vi "10-Tap 8-Bit Camera with DRAM (Host).vi"() -> ()   [LabVIEW 2014]
doc: "This is the host VI for the 10-Tap 8-Bit Camera with DRAM example. This example demonstrates how to acquire images from a 10-tap, 8-bit, extended configuration, Camera Link camera and display the images on the host. This example supports area scan and line scan cameras for both continuous and finite acquisitions.\n\nThis example also demonstrates the use of DRAM as a frame buffer for very high speed acquisitions. Data packing and flow-control are also employed to maximize use of the available DRAM and FIFOs in terms of both memory space and performance.\n\nAdditionally, the example demonstrates the serial server, which allows third-party camera configuration utilities to communicate with the camera using the Camera Link serial interface while this VI is running."
uses:
  <vilib>/userdefined/High Color/nirio_resource_hc.ctl
  <vilib>/FPGAPlugInAG/PCIe-1473R/niLvFpga_Open_PCIe-1473R.vi
  <vilib>/rvi/interface/common/dynamic/niFpgaDynamicAddResources.vi
  <vilib>/FPGAPlugInAG/Dynamic/niLvFpga_Reset_Dynamic.vi
  <vilib>/Utility/error.llb/Error Cluster From Error Code.vi
  <vilib>/rvi/errors/niLvFpgaAdjustHostInterfaceError.vi
  <vilib>/FPGAPlugInAG/Dynamic/niLvFpga_Run_Dynamic.vi
  <vilib>/rvi/interface/common/niFpgaWaitOnOcc.vi
  <vilib>/DAQmx/write.llb/DAQmx Write (Analog DBL 1Chan 1Samp).vi
  <vilib>/FPGAPlugInAG/Dynamic/niLvFpga_Close_Dynamic.vi
  <vilib>/rvi/interface/nirviOpenFPGA/nirviOpenFPGA.xnode
  FPGA Bitfiles/10-Tap8-bitCamer_FPGATarget_10-Tap8-bitCamer_C490DC32.lvbitx
  <vilib>/rvi/interface/nirviMethod/nirviMethod.xnode
  <vilib>/rvi/interface/nirviReadWriteControl/nirviReadWriteControl.xnode
  <vilib>/rvi/interface/nirviCloseFPGA/nirviCloseFPGA.xnode
  <vilib>/rvi/interface/Simulation/niFpgaSimulationCallBeginRW.vi
  <vilib>/rvi/errors/niLvFpgaMergeErrorWithErrorCode.vi
  NiFpgaLv.dll
  <vilib>/FPGAPlugInAG/Dynamic/niLvFpga_ConfigureFifo_Dynamic.vi
  <vilib>/FPGAPlugInAG/Dynamic/niLvFpga_StartFifo_Dynamic.vi
  <vilib>/FPGAPlugInAG/Dynamic/niLvFpga_ReadFifo_Dynamic.vi
  fish tracking dll/labview/find_fish_position.lvlib
  fish tracking dll/bin/find_fish_position.dll
panel:
  in  "Bin Threshold":i32=30
  in  "Axis Speed":dbl=50.0
  in  "Joystick":bool
  in  "Track":bool
  out "FISH_FOUND":bool
  in  "Bkg Image Path (must be the same size as the grabbed image)":path=path "C:/Users/Elizabeth/Desktop/bck_fish.png"
  in  "shift":i32
  in  "ROI_height":i32=180
  in  "ROI_witdth":i32=180
  out "Centroid":cluster{"y":i32, "x":i32}
  in  "SpeedFactor":dbl=1.0
  in  "offset":dbl(slide)=172.02643171806167 scale=150.0..250.0
  in  "Y_Target":dbl=219.0
  in  "X_Target":dbl=211.0
  out "TimeDelay":dbl=0.003333078930154443
  in  "setROI":bool=TRUE
  out "DstImageOpenCV":T1(plugin-control)
  in  "Esize_open":i32(slide)=4 scale=3.0..10.0
  in  "Esize_close":i32(slide)=4 scale=3.0..10.0
  in  "DMA Buffer Size\n(In Images)":u32=64 caption="DMA Buffer Size"
  in  "Signal Mapping":T2(ring)=enum."Basler 10-tap"
  out "Acq In Progress":bool=TRUE
  in  "Line Scan":bool
  in  "Frames To Acquire":u32 caption="Frames To Acquire\n(0 = infinite)"
  in  "Cancel":bool
  out "Acq'd Frame Width":u32=480
  in  "Stopped":bool=TRUE
  in  "RIO Device":T3="RIO0"
  out "DMA Write Timeout":bool
  in  "Start Serial Server":bool=TRUE
  out "Frames Acq'd":u32=128789
  out "Acq'd Frame Height":u32=400
  in  "Acquire":bool
  in  "Stop":bool
  in  "Image Height":u32=400 max=65535
  in  "Image Width":u32=480 max=65535 step=40
  out "Initialized":bool
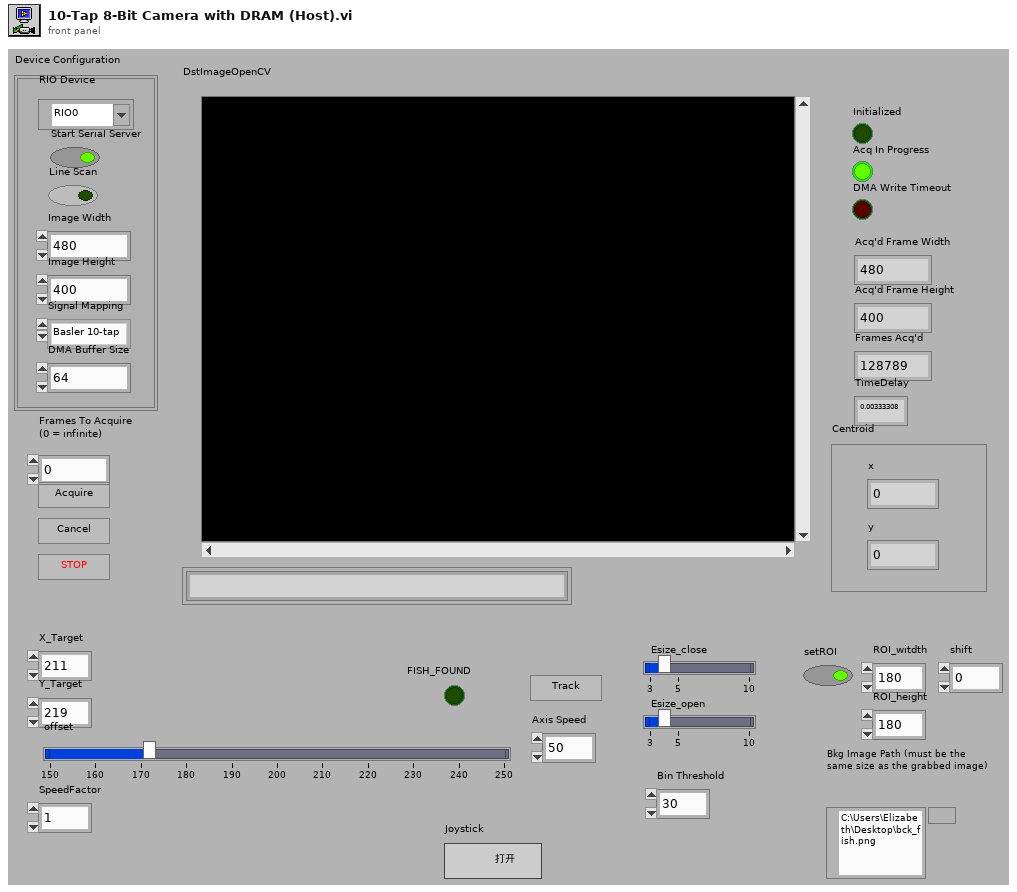
[diagram p1: front panel]
types:
  T1 = typedef "IMAQ Image.ctl" = refnum<image>
  T2 = enum8{"Standard", "Basler 10-tap", "Vosskühler 10-tap"}
  T3 = typedef "nirio_resource_hc.ctl" = tag
  T4 = typedef "Image Type" = u32
  T5 = enum16{"big-endian, network order", "native, host order", "little-endian"}
  T6 = enum32{"Invalid", "Standard", "Closed", "Hidden", "Minimized", "Maximized"}
  T7 = enum32{"Map Pixel Pointer", "Unmap Pixel Pointer", "Get Pixels Infos"}
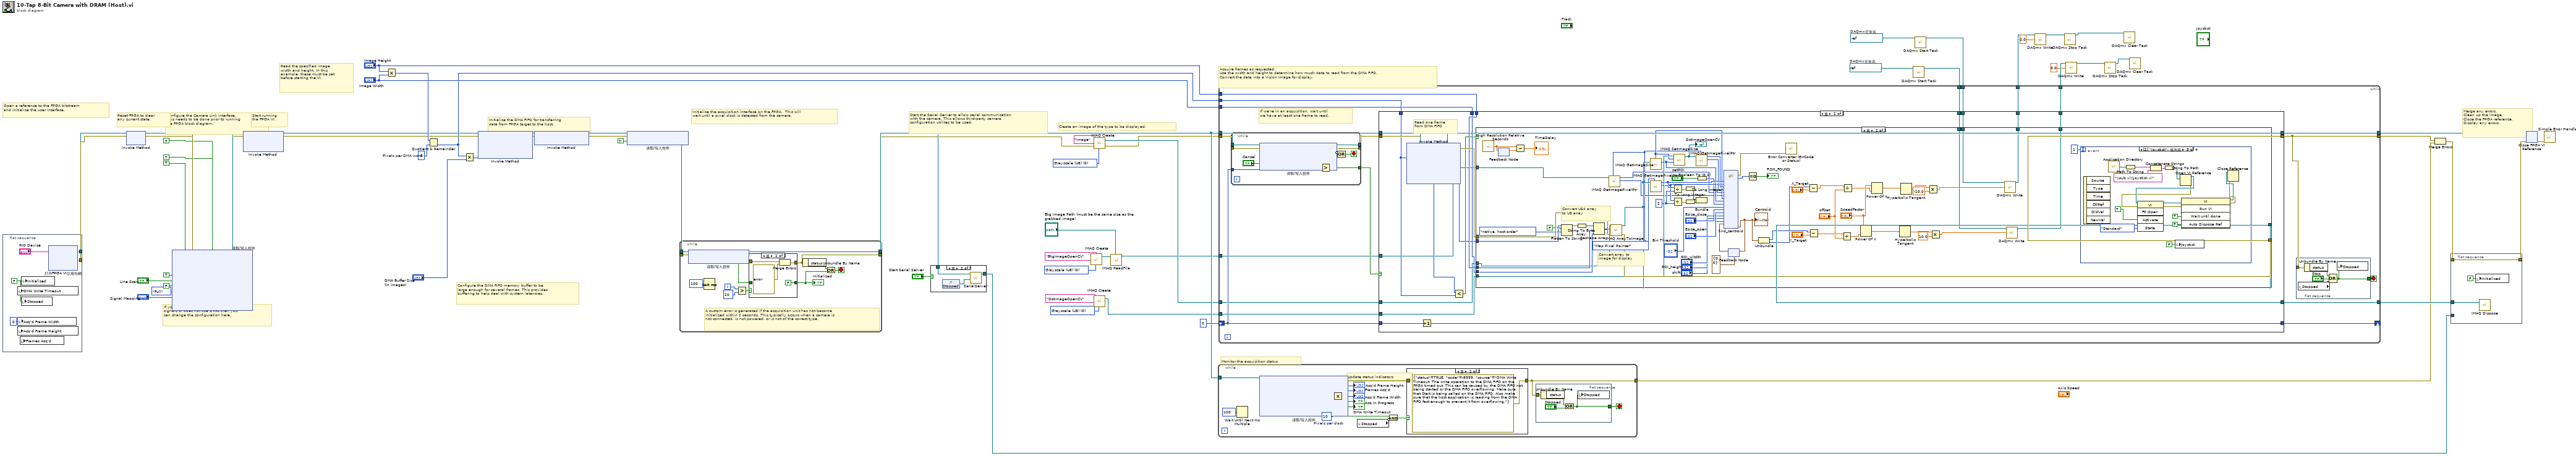
[diagram p0: block diagram]
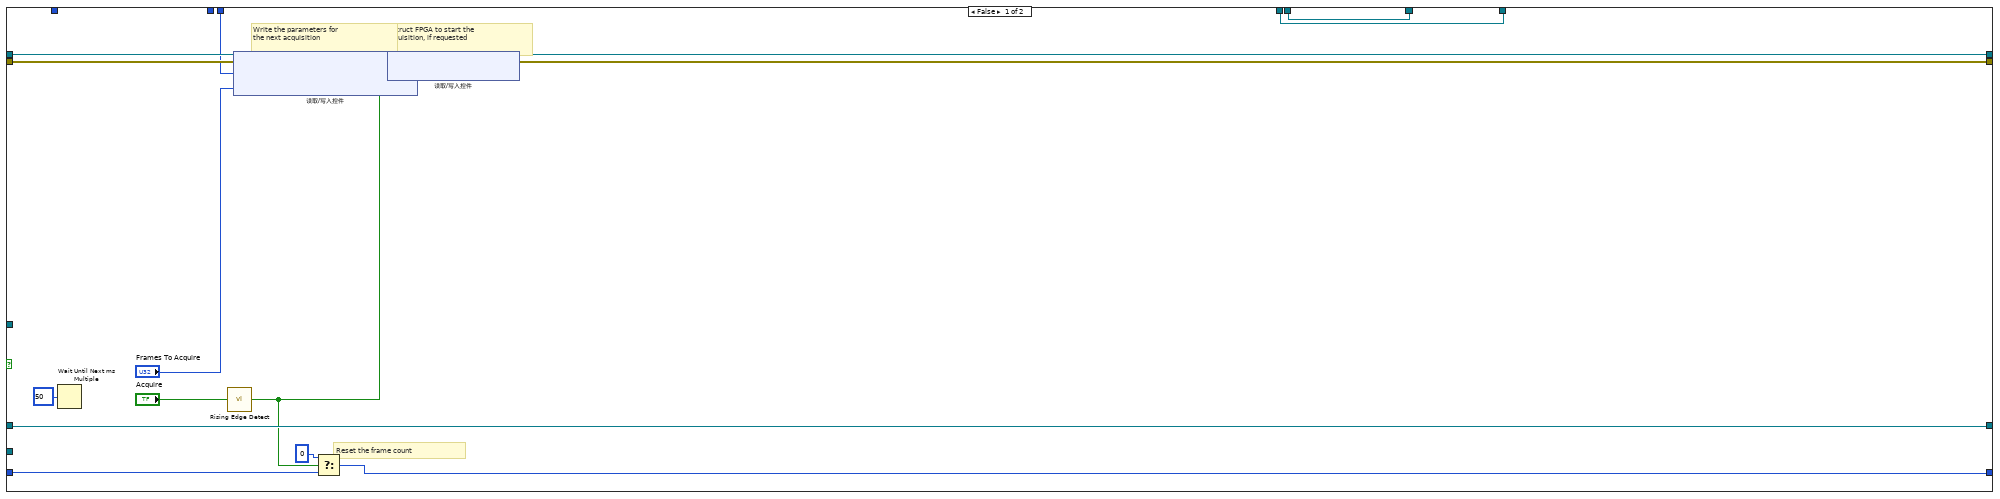
[diagram p4: hidden frame]
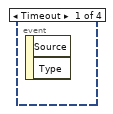
[diagram p6: hidden frame]
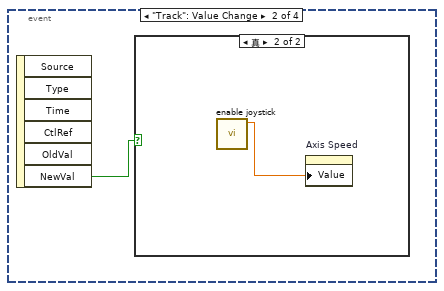
[diagram p7: hidden frame]
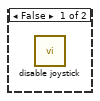
[diagram p8: hidden frame]
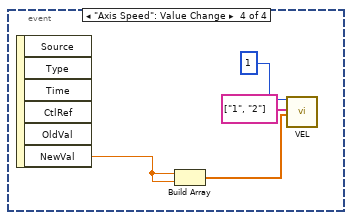
[diagram p9: hidden frame]
diagram:
  w2 = T4 0 items=["Grayscale (U8)", "Grayscale (I16)", "Grayscale (SGL)", "Complex (CSG)", "RGB (U32)", "HSL (U32)", "RGB (U64)", "Grayscale (U16)"] ("Image Type")
  w16 = refnum<k21> "Stage_Y"  # DAQmx任务名
  w17 = refnum<k21> "Stage_X"  # DAQmx任务名
  w19 = T4 0 items=["Grayscale (U8)", "Grayscale (I16)", "Grayscale (SGL)", "Complex (CSG)", "RGB (U32)", "HSL (U32)", "RGB (U64)", "Grayscale (U16)"] ("Image Type")
  w25 = u32 8  # Pixels per DMA word
  w62 = T4 0 items=["Grayscale (U8)", "Grayscale (I16)", "Grayscale (SGL)", "Complex (CSG)", "RGB (U32)", "HSL (U32)", "RGB (U64)", "Grayscale (U16)"] ("Image Type")
  # "If your camera outputs active-low enable\nsignals or does not use DVAL then you \ncan change the configuration here."
  # "Configure the DMA FIFO memory buffer to be\nlarge enough for several frames. This provides\nbuffering to help deal with system latencies."
  # "Start running\nthe FPGA VI."
  # "Reset FPGA to clear\nany current state."
  # "Read the specified image\nwidth and height. In this\nexample, these must be set\nbefore starting the VI."
  # "Merge any errors.\nClean up the image.\nClose the FPGA reference.\nDisplay any errors."
  # "Acquire frames as requested.\nUse the width and height to determine how much data to read from the DMA FIFO.\nConvert the data into a Vision Image for display."
  # "Monitor the acquisition status"
  # "Start the Serial Server to allow serial communication\nwith the camera. This allows third-party camera\nconfiguration utilites to be used."
  # "Create an image of the type to be displayed."
  # "Initialize the acquisition interface on the FPGA.  This will\nwait until a pixel clock is detected from the camera."
  # "Initialize the DMA FIFO for transferring\ndata from FPGA target to the host."
  # "Configure the Camera Link interface.\nThis needs to be done prior to running\nthe FPGA block diagram."
  # "Open a reference to the FPGA bitstream\nand initialize the user interface."
  n1 = flat-sequence {
    tunnel: [w68] -> w53
    tunnel: [w67] -> w66
    frame #0 {
      w71 = u32 0 ("Num Lines Acq'd")
      w70 = FALSE ("stop")
      n2 = local write "DMA Write Timeout"(w70) -> ()
      n3 = local write "Acq'd Frame Height"(w71) -> ()
      n4 = local write "Acq'd Frame Width"(w71) -> ()
      n5 = local write "Frames Acq'd"(w71) -> ()
      n6 = local write "Stopped"(w70) -> ()
      n7 = local write "Initialized"(w70) -> ()
      n8 = xnode "打开FPGA VI引用句柄"("资源名称"="RIO Device") -> ("FPGA VI引用输出"=w68:refnum<k20>, "错误输出"=w67:errorcluster)  [unwired: 1 in]
    }
  }
  n9 = xnode "Invoke Method"("FPGA VI引用输入"=w53, "错误输入"=w66) -> ("FPGA VI引用输出"=w42:refnum<k20>, "错误输出"=w45:errorcluster)
  n10 = xnode "读取/写入控件"("FPGA VI引用输入"=w42, "错误输入"=w45, "CL Config.FVAL Active High"=TRUE ("IO Module Config.CL FVAL Active High"), "CL Config.LVAL Active High"=TRUE ("IO Module Config.CL LVAL Active High"), "CL Config.DVAL Active High"=TRUE ("IO Module Config.CL DVAL Active High"), "CL Config.Spare Active High"=TRUE ("IO Module Config.CL Spare Active High"), "CL Config.Line Scan"="Line Scan", "Acq Control.Ignore DVAL"=FALSE ("CL Config.Line Scan"), "CL Config.Configuration"=enum8{"Base", "Medium", "Full"}."Full", "CL Config.Signal Mapping"="Signal Mapping") -> ("FPGA VI引用输出"=w46:refnum<k20>, "错误输出"=w44:errorcluster)
  n11 = xnode "Invoke Method"("FPGA VI引用输入"=w46, "错误输入"=w44) -> ("FPGA VI引用输出"=w22:refnum<k20>, "错误输出"=w21:errorcluster)  [unwired: 1 in]
  n12 = Multiply(x="Image Height", y="Image Width") -> (x*y=w24:u32)
  n13 = Quotient & Remainder(x=w24, y=w25) -> (floor(x/y)=w23:u32)  [unwired: 1 out]
  n14 = Multiply(x=w23, y="DMA Buffer Size\n(In Images)") -> (x*y=w36:u32)
  n15 = xnode "Invoke Method"("FPGA VI引用输入"=w22, "错误输入"=w21, "请求的深度"=w36) -> ("FPGA VI引用输出"=w52:refnum<k20>, "错误输出"=w51:errorcluster)  [unwired: 1 out]
  n16 = xnode "Invoke Method"("FPGA VI引用输入"=w52, "错误输入"=w51) -> ("FPGA VI引用输出"=w37:refnum<k20>, "错误输出"=w50:errorcluster)
  n17 = xnode "读取/写入控件"("FPGA VI引用输入"=w37, "错误输入"=w50, "Acq Control.Initialize"=TRUE ("Arm Acquisition")) -> ("FPGA VI引用输出"=w65:refnum<k20>, "错误输出"=w64:errorcluster)
  n18 = while {
    tunnel: w65 -> [w79]
    tunnel: w64 -> [w78]
    tunnel: [w77] -> w33
    tunnel: [w81] -> w32
    i -> [w73]
    stop <- w84 stop-if-true
    # "A custom error is generated if the acquisition unit has not become\ninitialized within 2 seconds. This typically occurs when a camera is\nnot connected, is not powered, or is not of the correct type."
    n19 = xnode "读取/写入控件"("FPGA VI引用输入"=w79, "错误输入"=w78) -> ("FPGA VI引用输出"=w77:refnum<k20>, "错误输出"=w76:errorcluster, "Acq Status.Initialized"=w75:bool)
    n20 = Wait (ms)(milliseconds to wait=u32 100) -> ()  [unwired: 1 out]
    n21 = Greater?(x=w73, y=20) -> (0:w74:bool)
    n22 = case shown="真" w74 {
      tunnel: [w86 FALSE] -> w80
      tunnel: w75 -> [w86 _]
      tunnel: w76 -> [w85 w88]
      tunnel: [w85 w90] -> w81
      frame False {
      }
      frame True {
        n23 = Merge Errors(w88, errorcluster {"status"=TRUE, "code"=-8999, "source"="Acquisition Initialization: This error typically occurs when a camera is not properly connected, is not powered, or is not of the correct type."} ("error in")) -> (w90:errorcluster)
      }
    }
    "Initialized" <- w80
    n24 = Unbundle By Name(w81) -> ("status"=w83:bool)
    n25 = Or(x=w83, y=w80) -> (x .or. y?=w84:bool)
  }
  n26 = case shown="真" "Start Serial Server" {
    tunnel: [_ w91] -> w54
    tunnel: w33 -> [_ w92]
    frame False {
    }
    frame True {
      n27 = control-ref of="Stopped"() -> (w93:refnum<vi>)
      n28 = call "SerialServer.vi"("Stop Refnum"=w93, "FPGA VI Reference In"=w92) -> ("FPGA VI Reference Out"=w91:refnum<k20>)  [unwired: 5 in]
    }
  }
  n29 = call "IMAQ Create"("Image Name"="BkgImageOpenCV", "Image Type"=w2) -> ("New Image"=w4:T1)  [unwired: 3 in, 1 out]
  n30 = call "IMAQ Create"("Image Name"="Image", "Image Type"=w62, "error in (no error)"=w32) -> ("New Image"=w29:T1, "error out"=w28:errorcluster)  [unwired: 2 in]
  n31 = call "IMAQ Create"("Image Name"="DstImageOpenCV", "Image Type"=w19) -> ("New Image"=w18:T1)  [unwired: 3 in, 1 out]
  n32 = call "IMAQ ReadFile"("File Path"="Bkg Image Path (must be the same size as the grabbed image)", "Image"=w4) -> ("Image Out"=w1:T1)  [unwired: 5 in, 4 out]
  n33 = while {
    tunnel: w33 -> [w104]
    tunnel: [w107] -> w47
    stop <- w106 stop-if-true
    w97 = u32 10  # Pixels per clock
    # "Update status indicators"
    n34 = Wait Until Next ms Multiple(millisecond multiple=u32 100) -> ()  [unwired: 1 out]
    n35 = xnode "读取/写入控件"("FPGA VI引用输入"=w104) -> ("错误输出"=w103:errorcluster, "Acq Status.Lines Per Frame"=→"Acq'd Frame Height":u32, "Acq Status.Frames Acq'd"=→"Frames Acq'd":u32, "Acq Status.Clocks Per Line"=w98:u32, "Acq Status.Acq In Progress"=→"Acq In Progress":bool, "Acq Status.DMA Write Timeout"=w95:bool)  [unwired: 1 in, 1 out]
    "DMA Write Timeout" <- w95
    n36 = Multiply(x=w98, y=w97) -> (x*y=→"Acq'd Frame Width":u32)
    n37 = local read "Stopped"() -> (w94:bool)
    n38 = Compound Arithmetic op=AND(w95, invert w94) -> (w96:bool)
    n39 = case shown="真" w96 {
      tunnel: w103 -> [w112 _]
      tunnel: [w112 errorcluster {"status"=TRUE, "code"=-8999, "source"="DMA Write Timeout: The write operation to the DMA FIFO on the FPGA timed out. This can be caused by the DMA FIFO not being started or the DMA FIFO overflowing. Make sure that Start is being called on the DMA FIFO. Also make sure that the host application is reading from the DMA FIFO fast enough to prevent it from overflowing."} ("error out")] -> w107
      frame False {
      }
      frame True {
      }
    }
    n40 = flat-sequence {
      tunnel: w107 -> [w111]
      tunnel: [w109] -> w106
      frame #0 {
        n41 = Unbundle By Name(w111) -> ("status"=w110:bool)
        n42 = Or(x=w110, y="Stopped") -> (x .or. y?=w109:bool)
        n43 = local write "Stopped"(w109) -> ()
      }
    }
  }
  n44 = call <vilib>:"DAQmx Start Task.vi"("task/channels in"=w16) -> ("task out"=w14:refnum<k21>)  [unwired: 13 in, 1 out]
  n45 = call <vilib>:"DAQmx Start Task.vi"("task/channels in"=w17) -> ("task out"=w15:refnum<k21>)  [unwired: 13 in, 1 out]
  n46 = while {
    tunnel: w33 -> [w126]
    tunnel: w28 -> [w125]
    tunnel: w23 -> [w134]
    tunnel: "Image Height" -> [w133]
    tunnel: "Image Width" -> [w132]
    tunnel: w29 -> [w131]
    tunnel: [w129] -> w48
    tunnel: [w130] -> w61
    tunnel: [w127] -> w56
    shift-right: [w121] -> _
    shift-left: u32 0 -> [w120]
    tunnel: w18 -> [w119]
    tunnel: w15 -> [w118]
    tunnel: w14 -> [w117]
    tunnel: [w116] -> w13
    tunnel: [w115] -> w12
    tunnel: w1 -> [w114]
    stop <- w128 stop-if-true
    # "If we're in an acquisition, wait until\nwe have at least one frame to read."
    n47 = while {
      tunnel: w126 -> [w141]
      tunnel: w125 -> [w140]
      tunnel: [w138] -> w124
      tunnel: [w139] -> w123
      tunnel: w120 -> [w144]
      tunnel: [w142] -> w122
      stop <- w143 stop-if-true
      n48 = xnode "读取/写入控件"("FPGA VI引用输入"=w141, "错误输入"=w140, "Acq Control.Cancel Acq"="Cancel") -> ("FPGA VI引用输出"=w139:refnum<k20>, "错误输出"=w138:errorcluster, "Acq Status.Acq In Progress"=w137:bool, "Acq Status.Frames Acq'd"=w136:u32)
      n49 = Greater?(x=w136, y=w144) -> (0:w142:bool)
      n50 = Compound Arithmetic op=OR(invert w137, w142) -> (w143:bool)
    }
    n51 = case shown="真" w122 {
      tunnel: w123 -> [w162 w180]
      tunnel: w124 -> [w161 w179]
      tunnel: w134 -> [_ w173]
      tunnel: w133 -> [w155 w187]
      tunnel: w132 -> [_ w186]
      tunnel: w131 -> [w166 w185]
      tunnel: [w157 w183] -> w129
      tunnel: [w160 w182] -> w130
      tunnel: [w166 w181] -> w127
      tunnel: w120 -> [w163 w178]
      tunnel: [w165 w177] -> w121
      tunnel: w119 -> [_ w172]
      tunnel: w118 -> [w151 w171]
      tunnel: w117 -> [w150 w170]
      tunnel: [w151 w169] -> w116
      tunnel: [w150 w168] -> w115
      tunnel: w114 -> [_ w167]
      frame False {
        # "Reset the frame count"
        # "Instruct FPGA to start the\nacquisition, if requested"
        # "Write the parameters for\nthe next acquisition"
        n52 = Wait Until Next ms Multiple(millisecond multiple=u32 50) -> ()  [unwired: 1 out]
        n53 = call "Rising Edge Detect.vi"("Input"="Acquire") -> ("Pulse"=w152:bool)  [unwired: 4 in]
        n54 = xnode "读取/写入控件"("FPGA VI引用输入"=w162, "错误输入"=w161, "Acq Control.Line Scan Height"=w155, "Acq Control.Frames To Acq"="Frames To Acquire") -> ("FPGA VI引用输出"=w159:refnum<k20>, "错误输出"=w158:errorcluster)
        n55 = Select(t=u32 0, s=w152, f=w163) -> (s? t:f=w165:u32)
        n56 = xnode "读取/写入控件"("FPGA VI引用输入"=w159, "错误输入"=w158, "Acq Control.Acquire"=w152) -> ("FPGA VI引用输出"=w160:refnum<k20>, "错误输出"=w157:errorcluster)
      }
      frame True {
        # "Read one frame\nfrom DMA FIFO"
        n57 = xnode "Invoke Method"("FPGA VI引用输入"=w180, "错误输入"=w179, "元素数量"=w173) -> ("FPGA VI引用输出"=w182:refnum<k20>, "错误输出"=w184:errorcluster, "数据"=w176:u64[], "剩余元素"=w174:u32)  [unwired: 1 in]
        n58 = Increment(x=w178) -> (x+1=w177:u32)
        n59 = Less?(x=w174, y=w173) -> (x < y?=w175:bool)
        n60 = case shown="真" w175 {
          tunnel: w187 -> [_ w260]
          tunnel: w186 -> [_ w259]
          tunnel: w185 -> [w191 w258]
          tunnel: w184 -> [w190 w257]
          tunnel: [w190 w256] -> w183
          tunnel: [w191 w249] -> w181
          tunnel: w176 -> [_ w253]
          tunnel: w172 -> [_ w248]
          tunnel: w171 -> [w189 w214]
          tunnel: w170 -> [w188 w213]
          tunnel: [w189 w212] -> w169
          tunnel: [w188 w211] -> w168
          tunnel: w167 -> [_ w199]
          frame False {
            # "Do not display the image if we're falling behind in the acquisition."
          }
          frame True {
            w247 = u64 2 ("y")
            w196 = T7."Map Pixel Pointer" ("Function")
            # "Convert U64 array\nto U8 array"
            # "Convert array to\nimage for display"
            n61 = call <vilib>:"High Resolution Relative Seconds.vi"() -> ("relative seconds"=w232:dbl)
            n62 = feedback-in #1(w232) -> ()
            n63 = feedback #1() -> (w233:dbl)  [unwired: 1 in]
            n64 = Subtract(x=w232, y=w233) -> (x-y=→"TimeDelay":dbl)
            n65 = Flatten To String(anything=w253, prepend array or string size? (T)=FALSE, byte order (0:big-endian, network order)=T5."native, host order") -> (data string=w251:string)  [unwired: 1 in, 2 out]
            n66 = String To Byte Array(string=w251) -> (unsigned byte array=w250:u8[])
            n67 = Reshape Array(w250, w260, w259) -> (w255:u8[][])
            n68 = call "IMAQ GetImagePixelPtr"("Function"=w196, "Image"=w199) -> ("LineWidth(Pixels)"=w197:i32, "Pixel Pointer out"=w198:u64)  [unwired: 4 in, 4 out]
            n69 = call "IMAQ ArrayToImage"("error in (no error)"=w257, "Image Pixels (U8)"=w255, "Image"=w258) -> ("error out"=w256:errorcluster, "Image Out"=w249:T1)  [unwired: 7 in]
            n70 = call "IMAQ GetImageSize"("Image"=w249) -> ("Y Resolution"=w239:i32, "X Resolution"=w240:i32)  [unwired: 3 in, 1 out]
            n71 = call "IMAQ GetImagePixelPtr"("Function"=w196, "Image"=w249) -> ("LineWidth(Pixels)"=w236:i32, "Pixel Pointer out"=w243:u64)  [unwired: 4 in, 4 out]
            n72 = Divide(x=w243, y=w247) -> (x/y=w246:dbl)
            n73 = Divide(x=w236, y=w247) -> (x/y=w245:dbl)
            n74 = call "IMAQ SetImageSize"("Y Resolution"=w239, "X Resolution"=w240, "Image"=w248) -> ("Image Out"=w244:T1)  [unwired: 2 in, 1 out]
            "DstImageOpenCV" <- w244
            n75 = To Long Integer(number=w246) -> (32bit integer=w210:i32)
            n76 = To Long Integer(number=w245) -> (32bit integer=w209:i32)
            n77 = call "IMAQ GetImagePixelPtr"("Function"=w196, "Image"=w244) -> ("LineWidth(Pixels)"=w241:i32, "Pixel Pointer out"=w242:u64)  [unwired: 4 in, 4 out]
            n78 = Boolean To (0,1)(Boolean="setROI") -> (0, 1=w235:i16)
            n79 = Bundle(w210, w209) -> ()  [unwired: 1 in, 1 out]
            n80 = feedback #2(cluster{"y":i32, "x":i32} {"y"=0, "x"=0} ("Centroid")) -> (w207:cluster{"y":i32, "x":i32})
            n81 = dll-call lib="C:/Users/Elizabeth/workspace/Tracking/TrackingUsingOpenCV - embedJoyStick/fish tracking dll/bin/find_fish_position.dll" fn="find_centroid"("ImagePtrSrc"=w243, "LineWidthSrc"=w236, "ImagePtrDst"=w242, "LineWidthDst"=w241, "ImagePtrBkg"=w198, "LineWidthBkg"=w197, "Width"=w240, "Height"=w239, "setROI"=w235, "BinThreshold"="Bin Threshold", "Esize_close"="Esize_close", "Esize_open"="Esize_open", "ROI_witdth"="ROI_witdth", "ROI_height"="ROI_height", "shift"="shift", "centroid_in"=w207) -> (error out=w200:errorcluster, "return type"=w194:i32, "Centroid"=w208:cluster{"y":i32, "x":i32})  [unwired: 20 in, 1 out]
            "Centroid" <- w208
            n82 = feedback-in #2(w208) -> ()
            n83 = Equal To 0?(x=w194) -> (x = 0?=→"FISH_FOUND":bool)
            n84 = Unbundle(w208) -> ("y"=w202:i32, "x"=w201:i32)
            n85 = call "Error Converter (ErrCode or Status).vi"("error in (no error)"=w200) -> ()  [unwired: 10 in, 1 out]
            n86 = Subtract(x=w201, y="X_Target") -> (x-y=w228:dbl)
            n87 = Subtract(x=w202, y="Y_Target") -> (x-y=w227:dbl)
            n88 = Divide(x=w227, y="offset") -> (x/y=w224:dbl)
            n89 = Divide(x=w228, y="offset") -> (x/y=w225:dbl)
            n90 = Power Of X(1:w224, 2:"SpeedFactor") -> (0:w221:dbl)
            n91 = Power Of X(1:w225, 2:"SpeedFactor") -> (0:w222:dbl)
            n92 = Hyperbolic Tangent(1:w221) -> (0:w217:dbl)
            n93 = Hyperbolic Tangent(1:w222) -> (0:w218:dbl)
            n94 = Multiply(x=w218, y=-10.0) -> (x*y=w216:dbl)
            n95 = Multiply(x=w217, y=10.0) -> (x*y=w215:dbl)
            n96 = call-poly <vilib>:"DAQmx Write.vi"("task/channels in"=w214, "data"=w216) -> ("task out"=w212:refnum<k21>)  [unwired: 11 in, 2 out]
            n97 = call-poly <vilib>:"DAQmx Write.vi"("task/channels in"=w213, "data"=w215) -> ("task out"=w211:refnum<k21>)  [unwired: 11 in, 2 out]
            n98 = event shown="[2] \"Joystick\": 值改变" {
              selector: _ -> [_ _ _ _]
              dyn-events: _ -> [_ _ _ _]
              timeout: 1 -> [_ _ _ _]
              event Timeout {
                n99 = event-data() -> ()  [unwired: 1 in, 2 out]
              }
              event "Track": Value Change {
                n100 = event-data() -> ("NewVal"=w261:bool)  [unwired: 1 in, 5 out]
                n101 = case shown="真" w261 {
                  frame False {
                    n102 = call "disable joystick.vi"() -> ()  [unwired: 12 in]
                  }
                  frame True {
                    n103 = call "enable joystick.vi"() -> ("元素"=w262:dbl)  [unwired: 11 in]
                    n104 = property on="Axis Speed" class="DigNum (严格)"("Value"=w262) -> ()  [unwired: 2 in, 2 out]
                  }
                }
              }
              event "Joystick": Value Change {
                n105 = event-data() -> ()  [unwired: 1 in, 6 out]
                n106 = call <vilib>:"Application Directory.vi"() -> ("Application Directory"=w278:path)
                n107 = Path To String(path=w278) -> (string=w277:string)
                n108 = Concatenate Strings(w277, "\\sub vi\\joystick.vi") -> (w275:string)
                n109 = String To Path(string=w275) -> (path=w274:path)
                n110 = local write "Joystick"(FALSE ("Joystick")) -> ()
                n111 = Open VI Reference(vi path=w274) -> (vi reference=w273:refnum<vi>, error out=w268:errorcluster)  [unwired: 5 in]
                n112 = invoke class="VI" method="FP.Open"(reference=w273, error in=w268, "Activate"=TRUE ("执行:调用时显示前面板"), "State"=T6."Standard" ("状态")) -> (reference out=w272:refnum<vi>, error out=w267:errorcluster)  [unwired: 1 in, 3 out]
                n113 = invoke class="VI" method="Run VI"(reference=w272, error in=w267, "Wait until done"=TRUE ("结束前等待"), "Auto Dispose Ref"=FALSE ("自动销毁引用")) -> (reference out=w269:refnum<vi>, error out=w266:errorcluster)  [unwired: 1 in, 3 out]
                n114 = Close Reference(reference=w269, error in (no error)=w266) -> ()  [unwired: 1 out]
              }
              event "Axis Speed": Value Change {
                n115 = event-data() -> ("NewVal"=w280:dbl)  [unwired: 1 in, 5 out]
                n116 = Build Array(w280, w280) -> (w281:dbl[])
                n117 = call "VEL.vi"("System no."=1, "Axes to set"=string[] ["1", "2"], "Velocity values"=w281) -> ()  [unwired: 15 in, 2 out]
              }
            }
          }
        }
      }
    }
    n118 = flat-sequence {
      tunnel: w129 -> [w147]
      tunnel: [w146] -> w128
      frame #0 {
        n119 = local read "Stopped"() -> (w145:bool)
        n120 = Unbundle By Name(w147) -> ("status"=w148:bool)
        n121 = Compound Arithmetic op=OR(w148, "Stop", w145) -> (w146:bool)
        n122 = local write "Stopped"(w146) -> ()
      }
    }
  }
  n123 = call-poly <vilib>:"DAQmx Write.vi"("task/channels in"=w13, "data"=0.0) -> ("task out"=w11:refnum<k21>)  [unwired: 11 in, 2 out]
  n124 = call <vilib>:"DAQmx Stop Task.vi"("task/channels in"=w11) -> ("task out"=w7:refnum<k21>)  [unwired: 13 in, 1 out]
  n125 = call-poly <vilib>:"DAQmx Write.vi"("task/channels in"=w12, "data"=0.0) -> ("task out"=w9:refnum<k21>)  [unwired: 11 in, 2 out]
  n126 = call <vilib>:"DAQmx Stop Task.vi"("task/channels in"=w9) -> ("task out"=w6:refnum<k21>)  [unwired: 13 in, 1 out]
  n127 = call <vilib>:"DAQmx Clear Task.vi"("task in"=w7) -> ()  [unwired: 14 in, 1 out]
  n128 = call <vilib>:"DAQmx Clear Task.vi"("task in"=w6) -> ()  [unwired: 14 in, 1 out]
  n129 = Merge Errors(w48, w47) -> (w49:errorcluster)
  n130 = flat-sequence {
    tunnel: w49 -> [w284]
    tunnel: [w284] -> w58
    tunnel: w56 -> [w285]
    tunnel: w54 -> [_]
    frame #0 {
      n131 = local write "Initialized"(FALSE ("Module Enabled")) -> ()
      n132 = call "IMAQ Dispose"("Image"=w285) -> ()  [unwired: 5 in, 1 out]
    }
  }
  n133 = xnode "Close FPGA VI Reference"("FPGA VI引用输入"=w61, "错误输入"=w58) -> ("错误输出"=w55:errorcluster)
  n134 = call <vilib>:"Simple Error Handler.vi"("error in (no error)"=w55) -> ()  [unwired: 4 in, 5 out]
